vi "用户登录.vi"() -> ()   [LabVIEW 2019]
panel:
  out "error out 3":errorcluster
  out "error out 2":errorcluster
  out "错误输出 4":errorcluster caption="错误输出"
  out "错误输出 3":errorcluster caption="错误输出"
  out "错误输出 2":errorcluster caption="错误输出"
  in  "用户类型":string(combo)="admin"
  out "错误输出":errorcluster
  in  "退出":bool
  in  "注册":bool
  in  "密   码":string
  in  "登录":bool
  in  "用户名":string
  out "Rows Fetched":i32
  out "error out":errorcluster
  out "Data":string[][](array[string])
  # "用户登录系统"
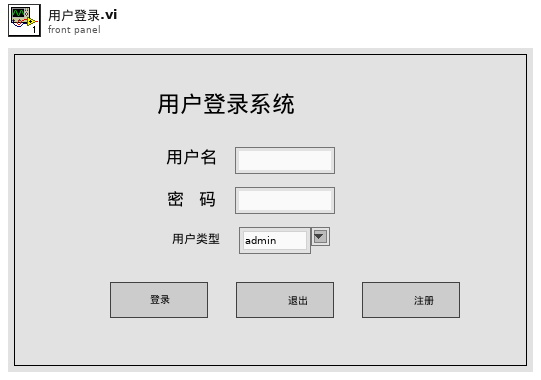
[diagram p1: front panel]
types:
  T1 = cluster{"Read Access":enum8{"Allowed", "Required", "None"}, "Write Access":enum8{"Allowed", "Required", "None"}}
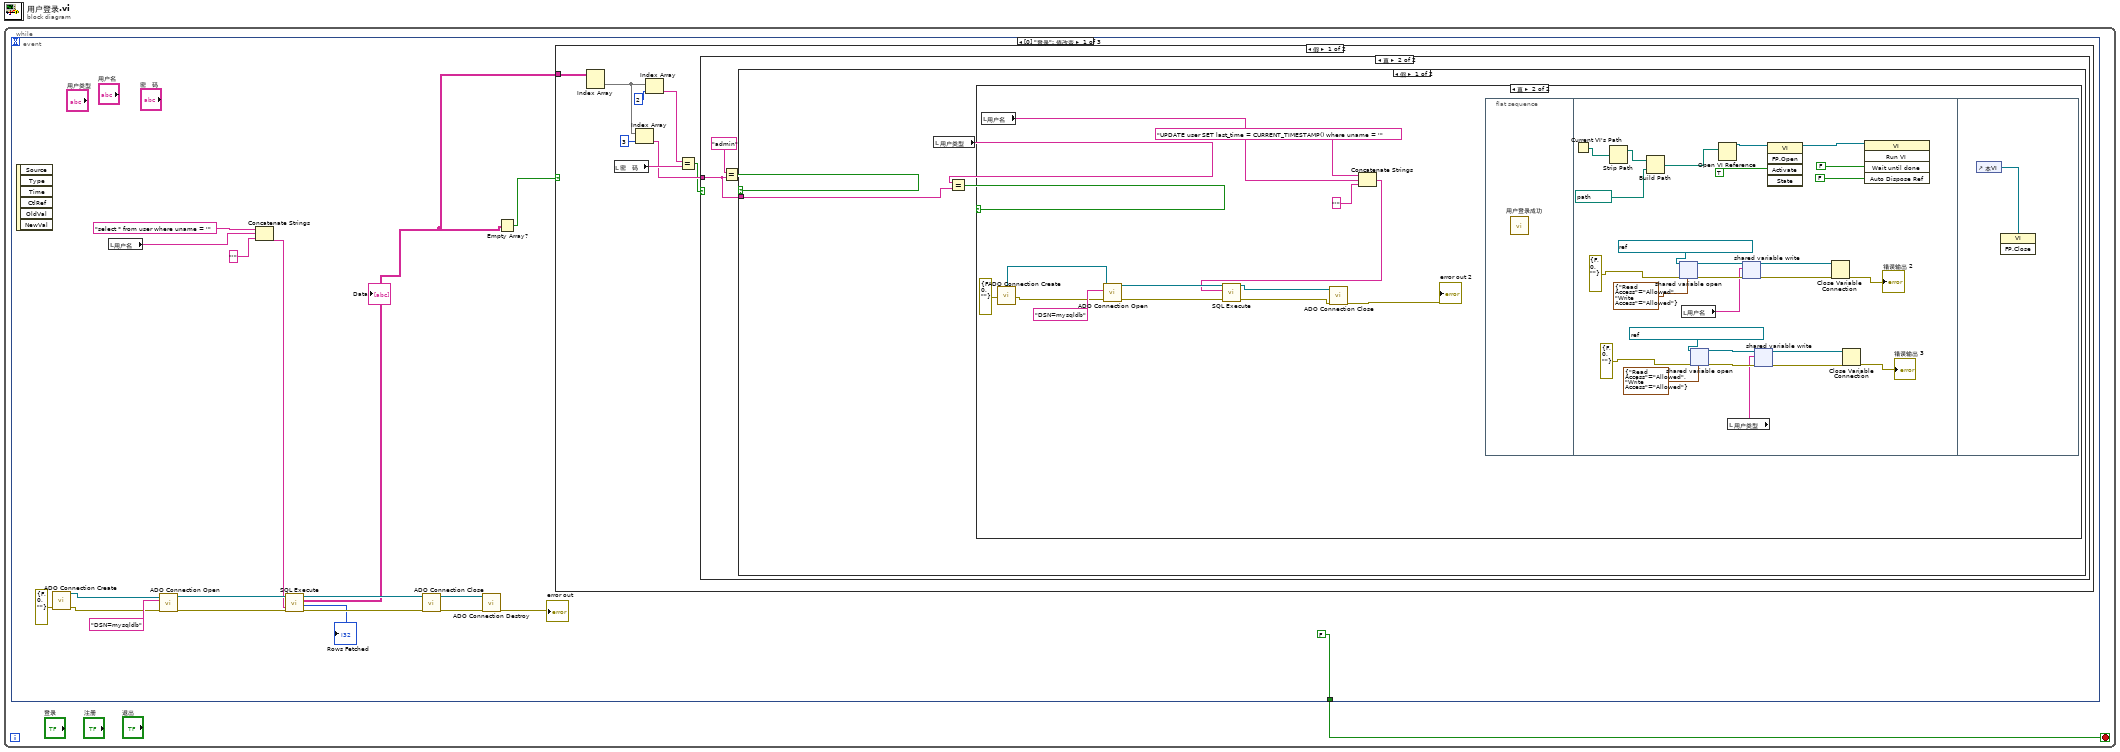
[diagram p0: block diagram]
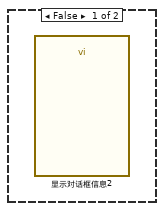
[diagram p2: hidden frame]
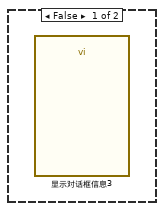
[diagram p3: hidden frame]
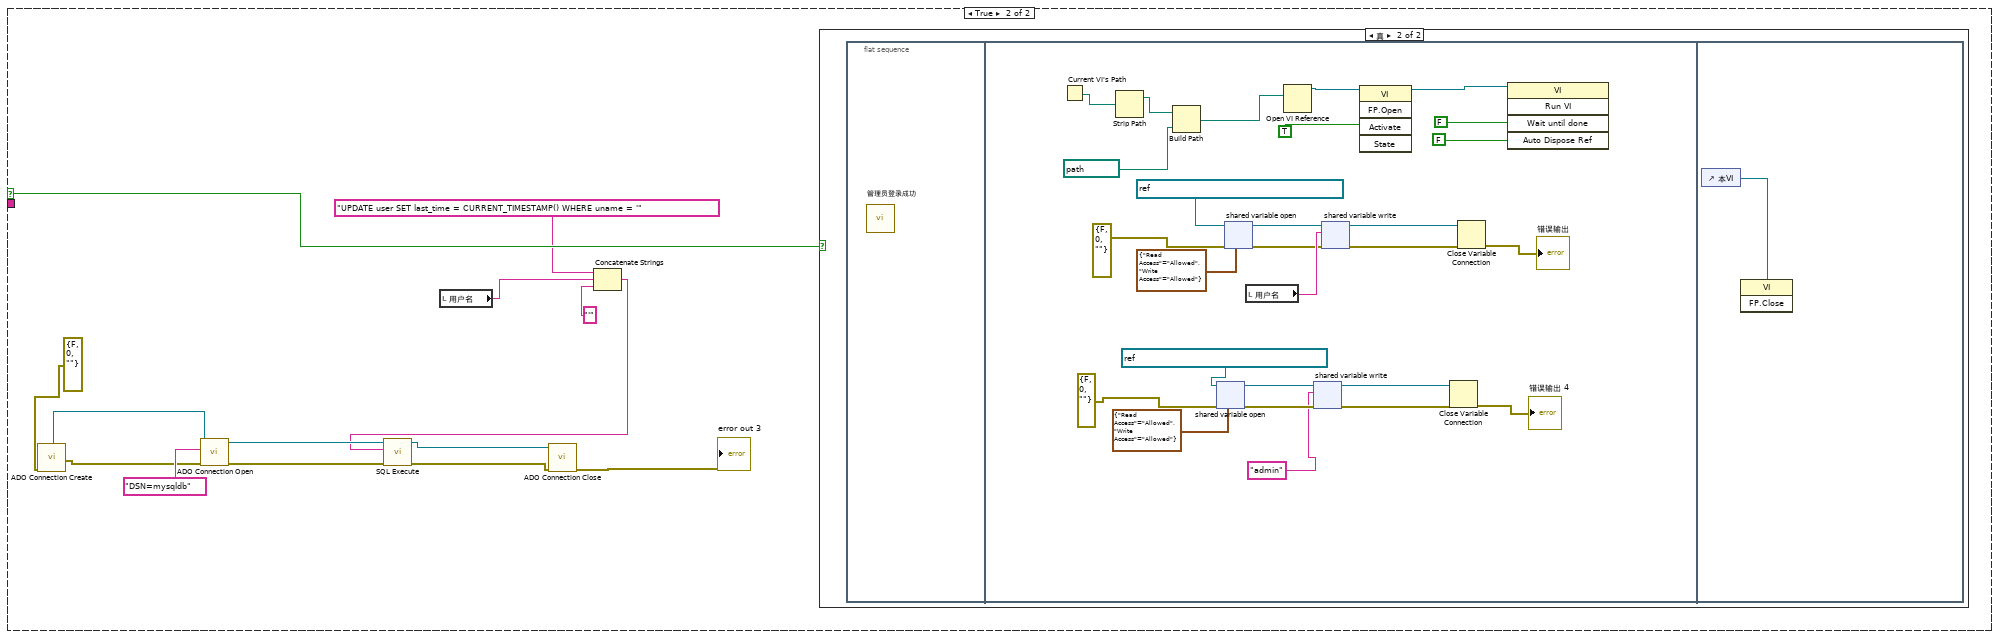
[diagram p4: hidden frame]
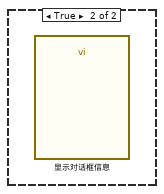
[diagram p6: hidden frame]
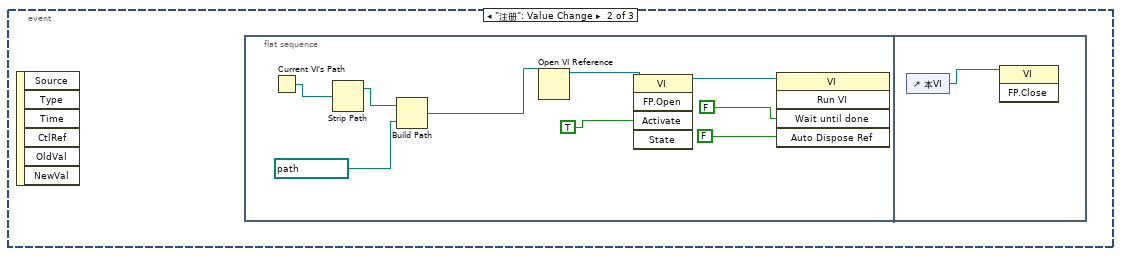
[diagram p7: hidden frame]
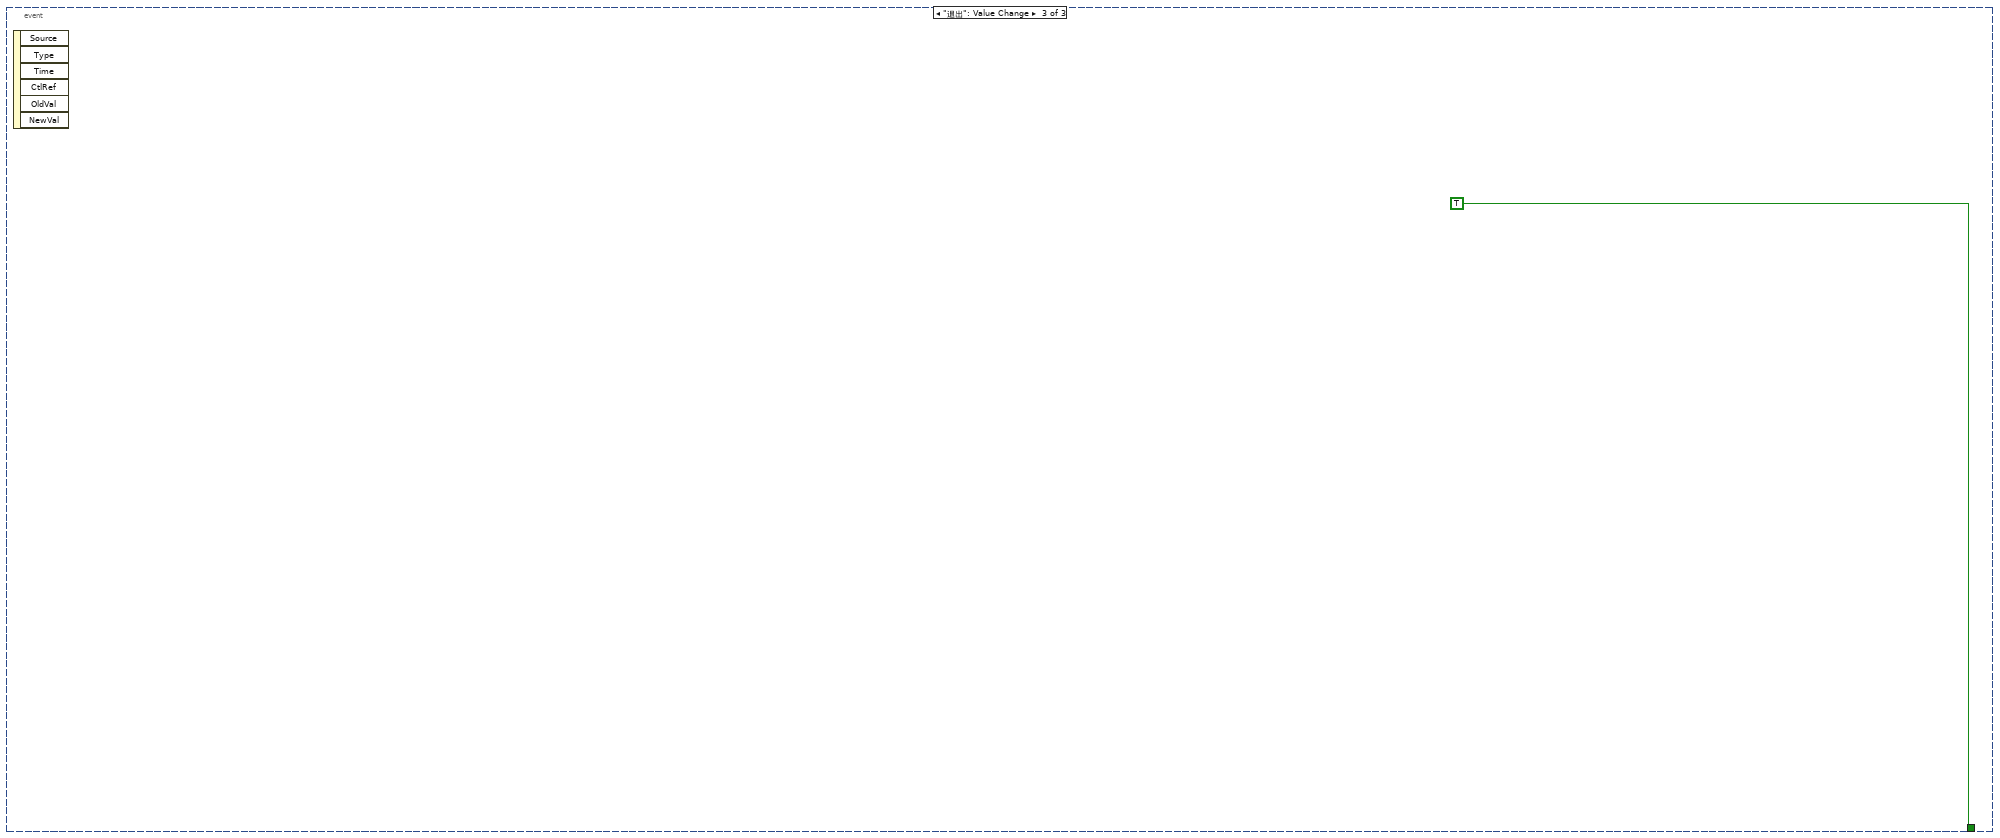
[diagram p8: hidden frame]
diagram:
  n1 = while {
    stop <- w1 stop-if-true
    n2 = event shown="[0] \"登录\": 值改变" {
      selector: _ -> [_ _ _]
      dyn-events: _ -> [_ _ _]
      timeout: _ -> [_ _ _]
      tunnel: [FALSE _ TRUE] -> w1
      event "登录": Value Change {
        n3 = event-data() -> ()  [unwired: 1 in, 6 out]
        n4 = call <userlib>:"ADO Connection Create.vi"("error in (no error)"=errorcluster {"status"=FALSE, "code"=0, "source"=""}) -> ("error out"=w16:errorcluster, "ADODB._Connection Out"=w20:refnum<k7>)  [unwired: 9 in]
        n5 = local read "用户名"() -> (w7:string)
        n6 = call <userlib>:"ADO Connection Open.vi"("error in (no error)"=w16, "ConnectionString"="DSN=mysqldb", "ADODB._Connection In"=w20) -> ("error out"=w15:errorcluster, "ADODB._Connection Out"=w19:refnum<k7>)  [unwired: 7 in]
        n7 = Concatenate Strings("select * from user where uname = '", w7, "'" ("字符串")) -> (w2:string)
        n8 = call <userlib>:"SQL Execute.vi"("error in (no error)"=w15, "Command Text"=w2, "ADODB._Connection In"=w19) -> ("error out"=w14:errorcluster, "Rows Fetched"=→"Rows Fetched":i32, "Data"=w5:string[][], "ADODB._Connection Out"=w18:refnum<k7>)  [unwired: 5 in]
        "Data" <- w5
        n9 = call <userlib>:"ADO Connection Close.vi"("error in (no error)"=w14, "ADODB._Connection In"=w18) -> ("error out"=w10:errorcluster, "ADODB._Connection Out"=w11:refnum<k7>)  [unwired: 8 in]
        n10 = call <userlib>:"ADO Connection Destroy.vi"("error in (no error)"=w10, "ADODB._Connection In"=w11) -> ("error out"=→"error out":errorcluster)  [unwired: 9 in]
        n11 = Empty Array?(array=w5) -> (empty?=w3:bool)
        n12 = case shown="假" w3 {
          tunnel: w5 -> [w28 _]
          frame False {
            n13 = Index Array(array=w28) -> (element=w21:string[])  [unwired: 2 in]
            n14 = local read "密   码"() -> (w26:string)
            n15 = Index Array(array=w21, index=3) -> (element=w24:string)
            n16 = Index Array(array=w21, index=2 ("索引")) -> (element=w22:string)
            n17 = Equal?(x=w22, y=w26) -> (x = y?=w23:bool)
            n18 = case shown="真" w23 {
              tunnel: w24 -> [_ w29]
              frame False {
                n19 = call "显示对话框信息2"() -> ()  [unwired: 10 in, 2 out]
              }
              frame True {
                n20 = Equal?(x="admin", y=w29) -> (x = y?=w30:bool)
                n21 = case shown="假" w30 {
                  selector: w30 -> [_ w89]
                  tunnel: w29 -> [w34 _]
                  frame False {
                    n22 = local read "用户类型"() -> (w33:string)
                    n23 = Equal?(x=w33, y=w34) -> (x = y?=w32:bool)
                    n24 = case shown="真" w32 {
                      frame False {
                        n25 = call "显示对话框信息3"() -> ()  [unwired: 10 in, 2 out]
                      }
                      frame True {
                        n26 = local read "用户名"() -> (w45:string)
                        n27 = call <userlib>:"ADO Connection Create.vi"("error in (no error)"=errorcluster {"status"=FALSE, "code"=0, "source"=""}) -> ("error out"=w42:errorcluster, "ADODB._Connection Out"=w44:refnum<k7>)  [unwired: 9 in]
                        n28 = call <userlib>:"ADO Connection Open.vi"("error in (no error)"=w42, "ConnectionString"="DSN=mysqldb", "ADODB._Connection In"=w44) -> ("error out"=w41:errorcluster, "ADODB._Connection Out"=w36:refnum<k7>)  [unwired: 7 in]
                        n29 = Concatenate Strings("UPDATE user SET last_time = CURRENT_TIMESTAMP() where uname = '", w45, "'" ("字符串")) -> (w35:string)
                        n30 = call <userlib>:"SQL Execute.vi"("error in (no error)"=w41, "Command Text"=w35, "ADODB._Connection In"=w36) -> ("error out"=w38:errorcluster, "ADODB._Connection Out"=w37:refnum<k7>)  [unwired: 5 in, 2 out]
                        n31 = call <userlib>:"ADO Connection Close.vi"("error in (no error)"=w38, "ADODB._Connection In"=w37) -> ("error out"=→"error out 2":errorcluster)  [unwired: 8 in, 1 out]
                        n32 = flat-sequence {
                          frame #0 {
                            n33 = call "用户登录成功"() -> ()  [unwired: 10 in, 2 out]
                          }
                          frame #1 {
                            n34 = Current VI's Path() -> (path=w69:path)
                            n35 = Strip Path(path=w69) -> (stripped path=w68:path)  [unwired: 1 out]
                            n36 = Build Path(base path=w68, name or relative path=path "登陆后.vi") -> (appended path=w66:path)
                            n37 = shared-variable-open(refnum<k21> "ni.var.psp://localhost/登录/登录用户" ("共享变量引用句柄输入"), errorcluster {"status"=FALSE, "code"=0, "source"=""} ("错误输入（无错误）"), T1 {"Read Access"=enum."Allowed", "Write Access"=enum."Allowed"} ("权限")) -> (w65:refnum<k21>, w62:errorcluster)
                            n38 = local read "用户名"() -> (w57:string)
                            n39 = shared-variable-open(refnum<k21> "ni.var.psp://localhost/登录/用户类型" ("共享变量引用句柄输入"), errorcluster {"status"=FALSE, "code"=0, "source"=""} ("错误输入（无错误）"), T1 {"Read Access"=enum."Allowed", "Write Access"=enum."Allowed"} ("权限")) -> (w56:refnum<k21>, w53:errorcluster)
                            n40 = Open VI Reference(vi path=w66) -> (vi reference=w70:refnum<vi>)  [unwired: 5 in, 1 out]
                            n41 = local read "用户类型"() -> (w48:string)
                            n42 = shared-variable-write(w65, w62, w57) -> (w64:refnum<k21>, w63:errorcluster)
                            n43 = shared-variable-write(w56, w53, w48) -> (w55:refnum<k21>, w54:errorcluster)
                            n44 = invoke class="VI" method="FP.Open"(reference=w70, "Activate"=TRUE) -> (reference out=w72:refnum<vi>)  [unwired: 3 in, 4 out]
                            n45 = Close Variable Connection(8:w63, 11:w64) -> (0:→"错误输出 2":errorcluster)
                            n46 = Close Variable Connection(8:w54, 11:w55) -> (0:→"错误输出 3":errorcluster)
                            n47 = invoke class="VI" method="Run VI"(reference=w72, "Wait until done"=FALSE, "Auto Dispose Ref"=FALSE) -> ()  [unwired: 2 in, 5 out]
                          }
                          frame #2 {
                            n48 = control-ref of="本VI"() -> (w75:refnum<vi>)
                            n49 = invoke class="VI" method="FP.Close"(reference=w75) -> ()  [unwired: 2 in, 3 out]
                          }
                        }
                      }
                    }
                  }
                  frame True {
                    n50 = call <userlib>:"ADO Connection Create.vi"("error in (no error)"=errorcluster {"status"=FALSE, "code"=0, "source"=""}) -> ("error out"=w84:errorcluster, "ADODB._Connection Out"=w86:refnum<k7>)  [unwired: 9 in]
                    n51 = call <userlib>:"ADO Connection Open.vi"("error in (no error)"=w84, "ConnectionString"="DSN=mysqldb", "ADODB._Connection In"=w86) -> ("error out"=w83:errorcluster, "ADODB._Connection Out"=w79:refnum<k7>)  [unwired: 7 in]
                    n52 = local read "用户名"() -> (w77:string)
                    n53 = Concatenate Strings("UPDATE user SET last_time = CURRENT_TIMESTAMP() WHERE uname = '", w77, "'" ("字符串")) -> (w78:string)
                    n54 = call <userlib>:"SQL Execute.vi"("error in (no error)"=w83, "Command Text"=w78, "ADODB._Connection In"=w79) -> ("error out"=w81:errorcluster, "ADODB._Connection Out"=w80:refnum<k7>)  [unwired: 5 in, 2 out]
                    n55 = call <userlib>:"ADO Connection Close.vi"("error in (no error)"=w81, "ADODB._Connection In"=w80) -> ("error out"=→"error out 3":errorcluster)  [unwired: 8 in, 1 out]
                    n56 = case shown="真" w89 {
                      frame False {
                      }
                      frame True {
                        n57 = flat-sequence {
                          frame #0 {
                            n58 = call "管理员登录成功"() -> ()  [unwired: 10 in, 2 out]
                          }
                          frame #1 {
                            n59 = Current VI's Path() -> (path=w111:path)
                            n60 = Strip Path(path=w111) -> (stripped path=w110:path)  [unwired: 1 out]
                            n61 = Build Path(base path=w110, name or relative path=path "登陆后.vi") -> (appended path=w108:path)
                            n62 = shared-variable-open(refnum<k21> "ni.var.psp://localhost/登录/用户类型" ("共享变量引用句柄输入"), errorcluster {"status"=FALSE, "code"=0, "source"=""} ("错误输入（无错误）"), T1 {"Read Access"=enum."Allowed", "Write Access"=enum."Allowed"} ("权限")) -> (w98:refnum<k21>, w95:errorcluster)
                            n63 = shared-variable-open(refnum<k21> "ni.var.psp://localhost/登录/登录用户" ("共享变量引用句柄输入"), errorcluster {"status"=FALSE, "code"=0, "source"=""} ("错误输入（无错误）"), T1 {"Read Access"=enum."Allowed", "Write Access"=enum."Allowed"} ("权限")) -> (w107:refnum<k21>, w102:errorcluster)
                            n64 = local read "用户名"() -> (w106:string)
                            n65 = Open VI Reference(vi path=w108) -> (vi reference=w112:refnum<vi>)  [unwired: 5 in, 1 out]
                            n66 = shared-variable-write(w98, w95, "admin") -> (w97:refnum<k21>, w96:errorcluster)
                            n67 = shared-variable-write(w107, w102, w106) -> (w104:refnum<k21>, w103:errorcluster)
                            n68 = invoke class="VI" method="FP.Open"(reference=w112, "Activate"=TRUE) -> (reference out=w114:refnum<vi>)  [unwired: 3 in, 4 out]
                            n69 = Close Variable Connection(8:w96, 11:w97) -> (0:→"错误输出 4":errorcluster)
                            n70 = Close Variable Connection(8:w103, 11:w104) -> (0:→"错误输出":errorcluster)
                            n71 = invoke class="VI" method="Run VI"(reference=w114, "Wait until done"=FALSE, "Auto Dispose Ref"=FALSE) -> ()  [unwired: 2 in, 5 out]
                          }
                          frame #2 {
                            n72 = control-ref of="本VI"() -> (w117:refnum<vi>)
                            n73 = invoke class="VI" method="FP.Close"(reference=w117) -> ()  [unwired: 2 in, 3 out]
                          }
                        }
                      }
                    }
                  }
                }
              }
            }
          }
          frame True {
            n74 = call "显示对话框信息"() -> ()  [unwired: 10 in, 2 out]
          }
        }
      }
      event "注册": Value Change {
        n75 = event-data() -> ()  [unwired: 1 in, 6 out]
        n76 = flat-sequence {
          frame #0 {
            n77 = Current VI's Path() -> (path=w121:path)
            n78 = Strip Path(path=w121) -> (stripped path=w120:path)  [unwired: 1 out]
            n79 = Build Path(base path=w120, name or relative path=path "注册用户.vi") -> (appended path=w118:path)
            n80 = Open VI Reference(vi path=w118) -> (vi reference=w122:refnum<vi>)  [unwired: 5 in, 1 out]
            n81 = invoke class="VI" method="FP.Open"(reference=w122, "Activate"=TRUE) -> (reference out=w123:refnum<vi>)  [unwired: 3 in, 4 out]
            n82 = invoke class="VI" method="Run VI"(reference=w123, "Wait until done"=FALSE, "Auto Dispose Ref"=FALSE) -> ()  [unwired: 2 in, 5 out]
          }
          frame #1 {
            n83 = control-ref of="本VI"() -> (w127:refnum<vi>)
            n84 = invoke class="VI" method="FP.Close"(reference=w127) -> ()  [unwired: 2 in, 3 out]
          }
        }
      }
      event "退出": Value Change {
        n85 = event-data() -> ()  [unwired: 1 in, 6 out]
      }
    }
  }
